vi "Document Tests - .vi"(8 "error in (no error)":errorcluster) -> (0 "error out":errorcluster)   [LabVIEW 2020]
uses:
  src/LabVIEW NPOI/Document/Document.lvclass
  src/LabVIEW NPOI/Document/Document.lvclass/Document.ctl
  src/LabVIEW NPOI/Document/Get FilePath.vi
  <vilib>/addons/_JKI Toolkits/Caraya/classes/Assert/Assert Equal Value and Type_Variant.vi
  <vilib>/addons/_JKI Toolkits/Caraya/classes/Assert/Assert Error.vi
  <vilib>/addons/_JKI Toolkits/Caraya/classes/Test/Test.lvclass
  <vilib>/addons/_JKI Toolkits/Caraya/classes/Assert/Assert.lvclass
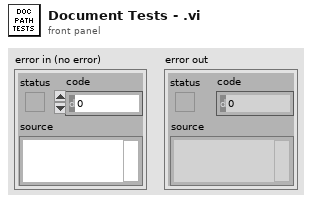
[diagram p1: front panel]
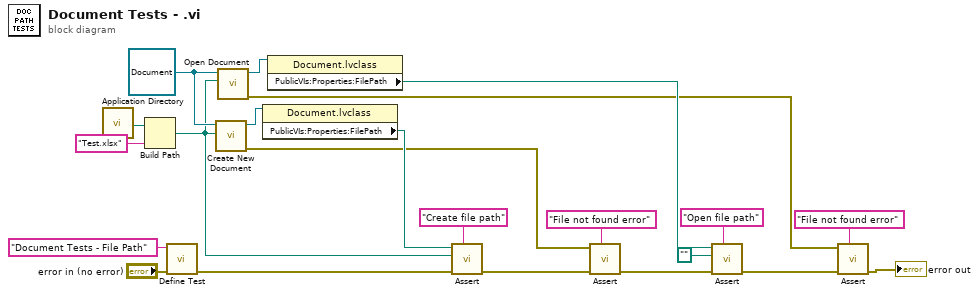
[diagram p0: block diagram]
diagram:
  w16 = refnum<class "Document.lvclass"> refnum ("Document in")
  n1 = call <vilib>:"Application Directory.vi"() -> ("Application Directory"=w15:path)
  n2 = Build Path(base path=w15, name or relative path="Test.xlsx" ("Label")) -> (appended path=w9:path)
  n3 = call <vilib>:"Define Test.vi"("error in (no error)"="error in (no error)", "Label (VI Title)"="Document Tests - File Path") -> ("error out"=w19:errorcluster)  [unwired: 9 in]
  n4 = call "Create New Document.vi"("File Path"=w9, "Document in"=w16) -> ("error out"=w2:errorcluster, "Document out"=w13:refnum<class "Document.lvclass">)  [unwired: 8 in]
  n5 = call "Open Document.vi"("File Path"=w9, "Document in"=w16) -> ("error out"=w3:errorcluster, "Document out"=w12:refnum<class "Document.lvclass">)  [unwired: 8 in]
  n6 = property class="Document.lvclass"(reference=w13) -> ("PublicVIs:Properties:FilePath"=w10:path)  [unwired: 1 in, 2 out]
  n7 = property class="Document.lvclass"(reference=w12) -> ("PublicVIs:Properties:FilePath"=w11:path)  [unwired: 1 in, 2 out]
  n8 = call-poly <vilib>:"Assert.vi"("Label"="Create file path", "error in (no error)"=w19, "Y"=w9, "X"=w10) -> ("error out"=w18:errorcluster)  [unwired: 7 in]
  n9 = call-poly <vilib>:"Assert.vi"("Label"="File not found error", "error in (no error)"=w18, "Error?"=w2) -> ("error out"=w8:errorcluster)  [unwired: 8 in]
  n10 = call-poly <vilib>:"Assert.vi"("Label"="Open file path", "error in (no error)"=w8, "Y"=path "", "X"=w11) -> ("error out"=w6:errorcluster)  [unwired: 7 in]
  n11 = call-poly <vilib>:"Assert.vi"("Label"="File not found error", "error in (no error)"=w6, "Error?"=w3) -> ("error out"=→"error out":errorcluster)  [unwired: 8 in]
